vi "createFAs.vi"(8 "error in (no error)":errorcluster, 11 "Boot in":refnum<class "Boot.lvclass">) -> (0 "error out":errorcluster, 2 "FAs":refnum<class "FAILC.lvclass">[](array[class]), 3 "Boot out":refnum<class "Boot.lvclass">)   [LabVIEW 2016, in "Boot.lvclass"]
uses:
  Boot.lvclass
  Common_RT_FAILC/FAILC/FAILC.lvclass
  Common_RT_FAILC/FAILCFactory/FAILCFactory.lvclass
  Common_RT_FAILC/DataTypes/FASettings.ctl
  Common_RT_ILC/DataTypes/ILCSettings.ctl
  Common_RT_FAILC/DataTypes/FATypes.ctl
  <vilib>/Utility/file.llb/Read Delimited Spreadsheet (string).vi
  Common_RT_ILC/RTILC.lvlib
  Common_RT_FAILC/RTFAILC.lvlib
panel:
  out "4":i32
  out "3":i32
  out "2":i32
  out "1":i32
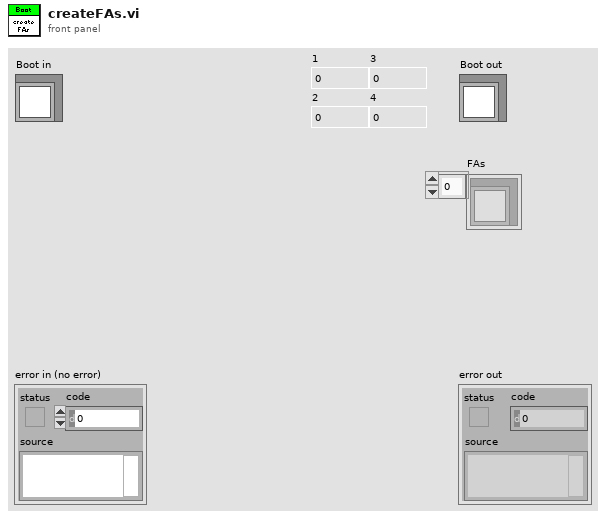
[diagram p1: front panel]
types:
  T1 = typedef "M1M3SupportSettings.lvlib/BaseILCSettings.ctl" = cluster{"CommunicationTimings":T2}
  T2 = typedef "RTILC.lvlib/ILCTimings.ctl" = cluster{"ReportServerID":u32, "ReportServerStatus":u32, "Mode":u32, "TemporaryAddress":u32, "Reset":u32, "ADCScanRate":u32, "ADCOffsetSensitivity":u32, "ReportCalibrationData":u32}
  T3 = typedef "M1M3SupportSettings.lvlib/BaseFASettings.ctl" = cluster{"CommunicationTimings":T4, "FATable":path}
  T4 = typedef "RTFAILC.lvlib/FATimings.ctl" = cluster{"BroadcastSetForce":u32, "BoosterValveGain":u32, "FreezeSensorValues":u32, "ForceAndStatus":u32, "ReadBoosterValveGain":u32, "SetForce":u32}
  T5 = typedef "RTFAILC.lvlib/FATypes.ctl" = enum16{"SingleAxis", "DualAxis"}
  T6 = typedef "RTFAILC.lvlib/FASettings.ctl" = cluster{"ILCSettings":T7, "ID":i16, "Type":T5, "XPosition":sgl, "YPosition":sgl, "ZPosition":sgl}
  T7 = typedef "RTILC.lvlib/ILCSettings.ctl" = cluster{"Subnet":u8, "Address":u8}
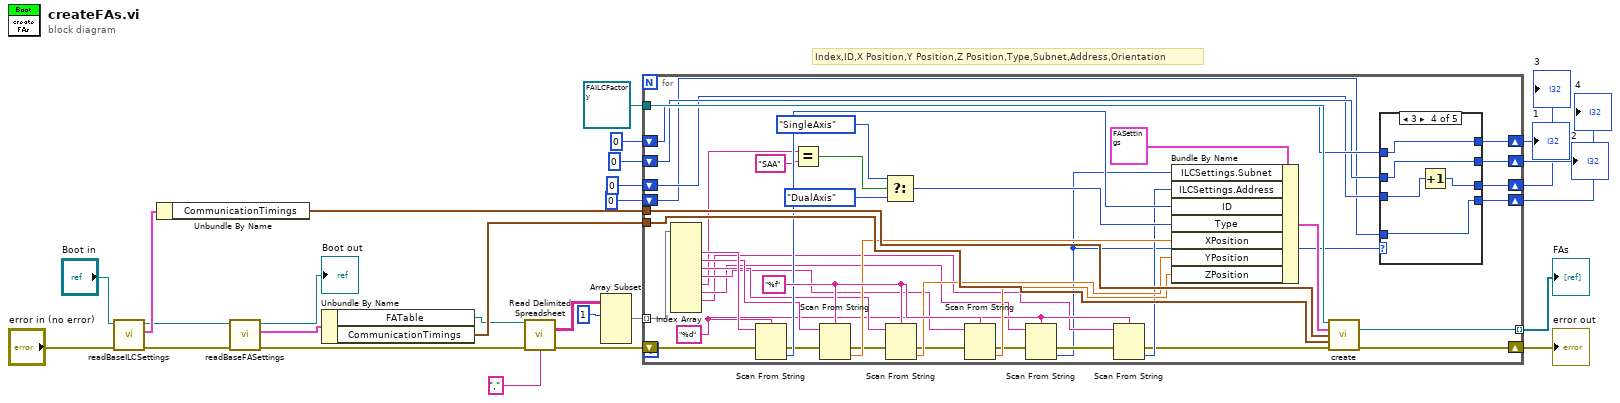
[diagram p0: block diagram]
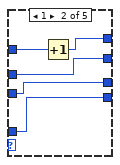
[diagram p3: hidden frame]
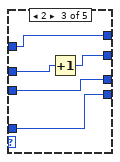
[diagram p4: hidden frame]
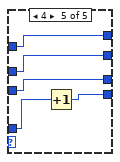
[diagram p5: hidden frame]
diagram:
  # "Index,ID,X Position,Y Position,Z Position,Type,Subnet,Address,Orientation"
  n1 = call "readBaseILCSettings.vi"("error in (no error)"="error in (no error)", "Boot in"="Boot in") -> ("error out"=w19:errorcluster, "BaseHardpointSettings"=w23:T1, "Boot out"=w20:refnum<class "Boot.lvclass">)  [unwired: 7 in]
  n2 = Unbundle By Name(w23) -> ("CommunicationTimings"=w22:T2)
  n3 = call "readBaseFASettings.vi"("error in (no error)"=w19, "Boot in"=w20) -> ("error out"=w11:errorcluster, "BaseForceActuatorSettings"=w17:T3, "Boot out"=→"Boot out":refnum<class "Boot.lvclass">)  [unwired: 7 in]
  n4 = Unbundle By Name(w17) -> ("FATable"=w12:path, "CommunicationTimings"=w26:T4)
  n5 = call-poly <vilib>:"Read Delimited Spreadsheet.vi"("file path (dialog if empty)"=w12, "error in (no error)"=w11, "delimiter (\\t)"="," ("delimiter (\\t)")) -> ("all rows"=w14:string[][], "error out"=w10:errorcluster)  [unwired: 7 in, 4 out]
  n6 = Array Subset(array=w14, index (row)=1 ("index")) -> (w9:string[][])  [unwired: 3 in]
  n7 = for {
    tunnel: refnum<class "FAILCFactory.lvclass"> refnum ("RTFAILC.lvlib:FAILCFactory.lvclass") -> [w65]
    shift-right: [w66] -> w27
    shift-left: w10 -> [w43]
    tunnel: w26 -> [w67]
    tunnel: w22 -> [w68]
    tunnel: [w64] -> w16 mode=indexing
    tunnel: w9 -> [w63] mode=indexing
    shift-right: [w34] -> w4
    shift-left: 0 -> [w35]
    shift-right: [w32] -> w3
    shift-left: 0 -> [w33]
    shift-right: [w30] -> w2
    shift-left: 0 -> [w31]
    shift-right: [w28] -> w1
    shift-left: 0 -> [w29]
    w47 = "%d" ("format string")
    w62 = "%f" ("format string")
    n8 = Index Array(array=w63) -> (element #2=w61:string, element #3=w59:string, element #4=w57:string, element #5=w55:string, element #6=w53:string, element #7=w46:string, element #8=w45:string)  [unwired: 9 in, 2 out]
    n9 = Scan From String(format string=w47, input string=w61, error in=w43) -> (error out=w42:errorcluster, output 1=w60:i32)  [unwired: 2 in, 2 out]
    n10 = Equal?(x=w53, y="SAA") -> (x = y?=w51:bool)
    n11 = Scan From String(format string=w62, input string=w59, error in=w42) -> (error out=w41:errorcluster, output 1=w58:dbl)  [unwired: 2 in, 2 out]
    n12 = Select(t=FATypes."SingleAxis" ("Type"), s=w51, f=FATypes."DualAxis") -> (s? t:f=w48:T5)
    n13 = Scan From String(format string=w62, input string=w57, error in=w41) -> (error out=w40:errorcluster, output 1=w56:dbl)  [unwired: 2 in, 2 out]
    n14 = Scan From String(format string=w62, input string=w55, error in=w40) -> (error out=w39:errorcluster, output 1=w54:dbl)  [unwired: 2 in, 2 out]
    n15 = Scan From String(format string=w47, input string=w46, error in=w39) -> (error out=w38:errorcluster, output 1=w36:i32)  [unwired: 2 in, 2 out]
    n16 = Scan From String(format string=w47, input string=w45, error in=w38) -> (error out=w37:errorcluster, output 1=w44:i32)  [unwired: 2 in, 2 out]
    n17 = Bundle By Name(cluster=T6 {"ILCSettings"={"Subnet"=0, "Address"=0}, "ID"=0, "Type"=enum."SingleAxis", "XPosition"=0.0, "YPosition"=0.0, "ZPosition"=0.0} ("FASettings"), "ILCSettings.Subnet"=w36, "ILCSettings.Address"=w44, "ID"=w60, "Type"=w48, "XPosition"=w58, "YPosition"=w56, "ZPosition"=w54) -> (w69:T6)
    n18 = call "create.vi"("FAILCFactory in"=w65, "FASettings"=w69, "ILCTimings"=w68, "FATimings"=w67, "error in (no error)"=w37) -> ("ForceActuator"=w64:refnum<class "FAILC.lvclass">, "error out"=w66:errorcluster)  [unwired: 8 in, 1 out]
    n19 = case shown="3" w36 {
      tunnel: w35 -> [w74 w79 w84 w89 w94]
      tunnel: [w74 w78 w84 w89 w94] -> w34
      tunnel: w33 -> [w73 w77 w83 w88 w93]
      tunnel: [w73 w77 w82 w88 w93] -> w32
      tunnel: w31 -> [w72 w76 w81 w87 w92]
      tunnel: [w72 w76 w81 w86 w92] -> w30
      tunnel: w29 -> [w71 w75 w80 w85 w91]
      tunnel: [w71 w75 w80 w85 w90] -> w28
      frame 0, Default {
      }
      frame 1 {
        n20 = Increment(x=w79) -> (x+1=w78:i32)
      }
      frame 2 {
        n21 = Increment(x=w83) -> (x+1=w82:i32)
      }
      frame 3 {
        n22 = Increment(x=w87) -> (x+1=w86:i32)
      }
      frame 4 {
        n23 = Increment(x=w91) -> (x+1=w90:i32)
      }
    }
  }
  "error out" <- w27
  "FAs" <- w16
  "1" <- w4
  "2" <- w3
  "3" <- w2
  "4" <- w1
